vi "Periodic Tasks.vi"(8 "error in":errorcluster) -> ()   [LabVIEW 2016]
doc: "This VI runs in parallel to other robot code. It can contain as many user-defined periodic loops as you need. These can carry out PID or other sorts of timed response."
uses:
  <vilib>/Rock Robotics/WPI/Utilities/WPI_GetSetVariantRefNum.vi
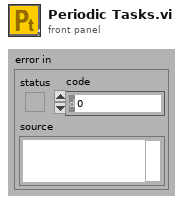
[diagram p1: front panel]
types:
  T1 = typedef "WPI_JoystickDevRef.ctl" = cluster{"Device":T2}
  T2 = typedef "WPI_JoystickDeviceEnum.ctl" = enum16{"USB 0", "USB 1", "USB 2", "USB 3", "USB 4", "USB 5"}
  T3 = typedef "WPI_EncoderDevRef.ctl" = cluster{"DevStatus":errorcluster, "EncoderIndex":T4, "CounterIndex":T5, "DistancePerCount":dbl, "Decoding Type":T6}
  T4 = typedef "FPGA_EncoderIdx.ctl" = enum8{"Enc 0", "Enc 1", "Enc 2", "Enc 3", "Enc 4", "Enc 5", "Enc 6", "Enc 7", "Invalid"}
  T5 = typedef "FPGA_CounterCtrSystemIndex.ctl" = enum8{"Ctr 0", "Ctr 1", "Ctr 2", "Ctr 3", "Ctr 4", "Ctr 5", "Ctr 6", "Ctr 7", "Invalid"}
  T6 = typedef "WPI_EncoderType.ctl" = enum16{"1x", "2x", "4x"}
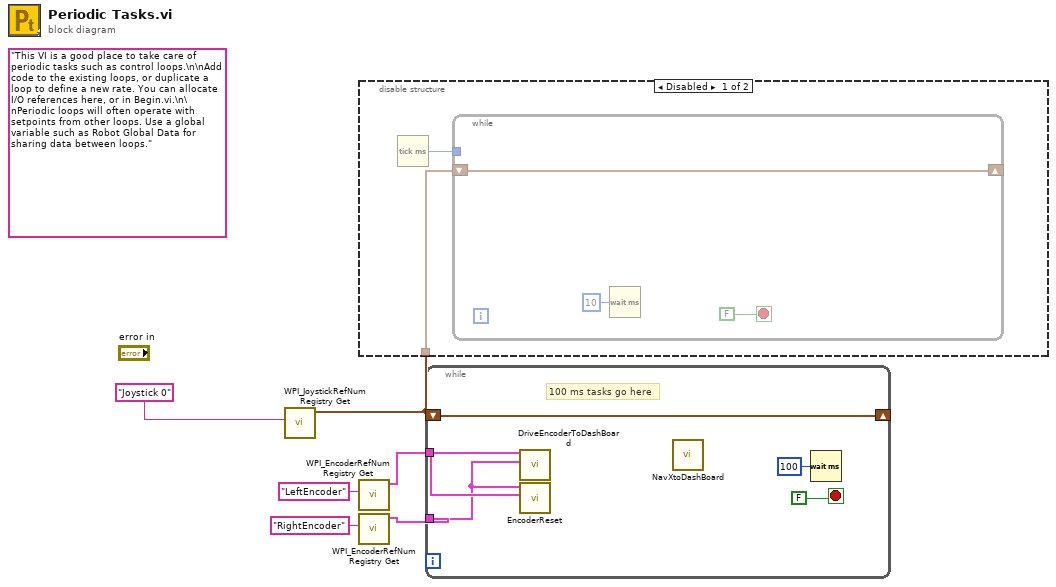
[diagram p0: block diagram]
diagram:
  (unwired) "This VI is a good place to take care of periodic tasks such as control loops.\n\nAdd code to the existing loops, or duplicate a loop to define a new rate. You can allocate I/O references here, or in Begin.vi.\n\nPeriodic loops will often operate with setpoints from other loops. Use a global variable such as Robot Global Data for sharing data between loops."
  n1 = call <vilib>:"WPI_JoystickRefNum Registry Get.vi"("refnum name"="Joystick 0") -> ("JoystickDevRef"=w5:T1)  [unwired: 1 in, 9 out]
  n2 = call <vilib>:"WPI_EncoderRefNum Registry Get.vi"("refnum name"="LeftEncoder") -> ("EncoderDevRef"=w1:T3)  [unwired: 9 in, 1 out]
  n3 = call <vilib>:"WPI_EncoderRefNum Registry Get.vi"("refnum name"="RightEncoder") -> ("EncoderDevRef"=w2:T3)  [unwired: 9 in, 1 out]
  n4 = disable-structure shown="Disabled" {
    disable-tunnel: w5 -> [w8 _]
    frame Disabled {
      n5 = Tick Count (ms)() -> (millisecond timer value=w7:u32)
      n6 = while {
        shift-right: [w10] -> _
        shift-left: w8 -> [w10]
        tunnel: w7 -> [_]
        stop <- FALSE stop-if-true
        n7 = Wait (ms)(milliseconds to wait=u32 10) -> ()  [unwired: 1 out]
      }
    }
    frame Enabled {
    }
  }
  n8 = while {
    shift-right: [w14] -> _
    shift-left: w5 -> [w14]
    tunnel: w2 -> [w12]
    tunnel: w1 -> [w13]
    stop <- FALSE stop-if-true
    # "100 ms tasks go here"
    n9 = call "DriveEncoderToDashBoard.vi"("EncoderDevRef"=w12, "EncoderDevRef 2"=w13) -> ()  [unwired: 10 in]
    n10 = call "EncoderReset.vi"("EncoderDevRef 2"=w13, "EncoderDevRef"=w12) -> ()  [unwired: 10 in]
    n11 = call "NavXtoDashBoard.vi"() -> ()  [unwired: 12 in]
    n12 = Wait (ms)(milliseconds to wait=u32 100) -> ()  [unwired: 1 out]
  }
